vi "_PC_Pub writeListboxString.vi"(5 "Reset (F)":bool, 6 "Display Error Msg? (F)":bool, 7 "String Color":u32(colorbox), 8 "error in (no error)":errorcluster, 10 "update_Str":string, 11 "Listbox Ref Input":refnum<vi>) -> (0 "error out":errorcluster, 3 "Listbox Ref Output":refnum<vi>)   [LabVIEW 2018]
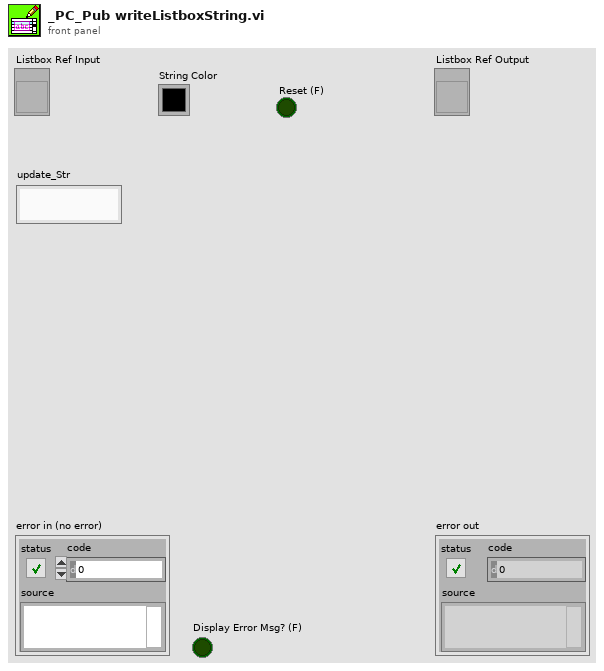
[diagram p1: front panel]
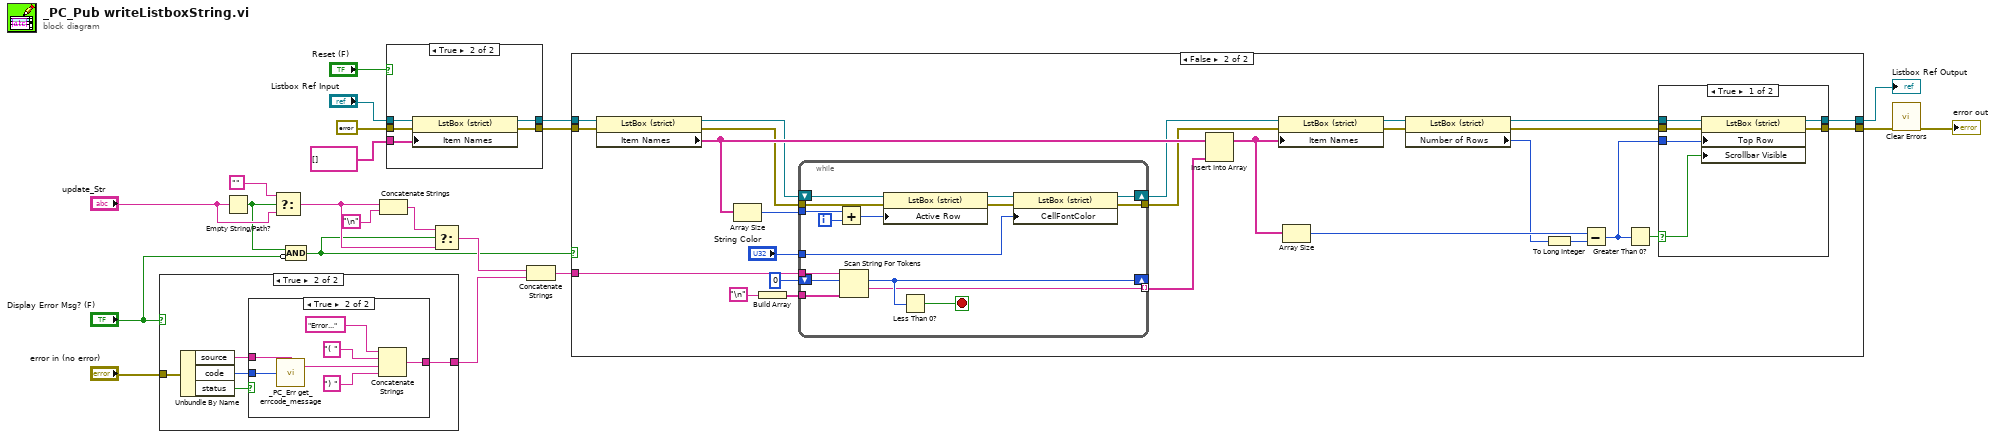
[diagram p0: block diagram]
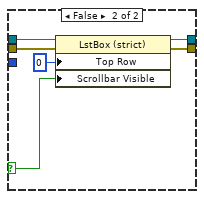
[diagram p3: hidden frame]
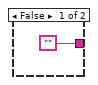
[diagram p5: hidden frame]
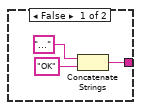
[diagram p6: hidden frame]
diagram:
  n1 = case shown="True" "Display Error Msg? (F)" {
    tunnel: "error in (no error)" -> [_ w27]
    tunnel: ["" w25] -> w21
    frame False {
    }
    frame True {
      n2 = Unbundle By Name(w27) -> ("source"=w23:string, "code"=w24:i32, "status"=w26:bool)
      n3 = case shown="True" w26 {
        tunnel: [w28 w35] -> w25
        tunnel: w24 -> [_ w33]
        tunnel: w23 -> [_ w31]
        frame False {
          n4 = Concatenate Strings("...", "OK") -> (w28:string)
        }
        frame True {
          n5 = call "_PC_Err get_errcode_message.vi"("err code"=w33, "sourceError"=w31) -> ("err msg"=w32:string)  [unwired: 1 out]
          n6 = Concatenate Strings("Error...", "( " ("string"), w32, ") " ("string")) -> (w35:string)
        }
      }
    }
  }
  n7 = Empty String/Path?(string/path="update_Str") -> (empty?=w11:bool)
  n8 = Select(t="", s=w11, f="update_Str") -> (s? t:f=w9:string)
  n9 = Compound Arithmetic op=AND(w11, invert "Display Error Msg? (F)") -> (w6:bool)
  n10 = Concatenate Strings(w9, "\n") -> (w8:string)
  n11 = case shown="True" "Reset (F)" {
    tunnel: "Listbox Ref Input" -> [w39 w44]
    tunnel: [w39 w43] -> w18
    tunnel: string[] [] ("appended array") -> [_ w42]
    tunnel: errorcluster {"status"=FALSE, "code"=0, "source"=""} ("error in (no error)") -> [w38 w41]
    tunnel: [w38 w40] -> w15
    frame False {
    }
    frame True {
      n12 = property class="LstBox (strict)"(reference=w44, error in=w41, "Item Names"=w42) -> (reference out=w43:refnum<vi>, error out=w40:errorcluster)
    }
  }
  n13 = Select(t=w8, s=w6, f=w9) -> (s? t:f=w7:string)
  n14 = Concatenate Strings(w7, w21) -> (w14:string)
  n15 = case shown="False" w6 {
    tunnel: w14 -> [_ w72]
    tunnel: w18 -> [w46 w68]
    tunnel: [w46 w60] -> w4
    tunnel: [w45 w59] -> w1
    tunnel: w15 -> [w45 w62]
    frame True {
    }
    frame False {
      n16 = property class="LstBox (strict)"(reference=w68, error in=w62) -> (reference out=w53:refnum<vi>, error out=w52:errorcluster, "Item Names"=w58:string[])
      n17 = Array Size(array=w58) -> (size(s)=w54:i32)
      n18 = Build Array("\n") -> (w71:string[])
      n19 = while {
        tunnel: w72 -> [w100]
        tunnel: w71 -> [w95]
        tunnel: [w96] -> w64 mode=indexing
        shift-right: [w99] -> _
        shift-left: 0 -> [w98]
        tunnel: w54 -> [w92]
        tunnel: w52 -> [w93]
        shift-right: [w87] -> w51
        shift-left: w53 -> [w94]
        tunnel: [w86] -> w50
        tunnel: "String Color" -> [w85]
        i -> [w91]
        stop <- w97 stop-if-true
        n20 = Add(x=w92, y=w91) -> (x+y=w90:i32)
        n21 = Scan String For Tokens(6:w95, 8:w98, 9:w100) -> (1:w96:string, 2:w99:i32)  [unwired: 3 in, 2 out]
        n22 = property class="LstBox (strict)"(reference=w94, error in=w93, "Active Row"=w90) -> (reference out=w89:refnum<vi>, error out=w88:errorcluster)
        n23 = Less Than 0?(x=w99) -> (x < 0?=w97:bool)
        n24 = property class="LstBox (strict)"(reference=w89, error in=w88, "CellFontColor"=w85) -> (reference out=w87:refnum<vi>, error out=w86:errorcluster)
      }
      n25 = Insert Into Array(array=w58, new element=w64) -> (w63:string[])  [unwired: 1 in]
      n26 = property class="LstBox (strict)"(reference=w51, error in=w50, "Item Names"=w63) -> (reference out=w48:refnum<vi>, error out=w47:errorcluster)
      n27 = Array Size(array=w63) -> (size(s)=w61:i32)
      n28 = property class="LstBox (strict)"(reference=w48, error in=w47) -> (reference out=w57:refnum<vi>, error out=w56:errorcluster, "Number of Rows"=w55:u32)
      n29 = To Long Integer(number=w55) -> (32bit integer=w67:i32)
      n30 = Subtract(x=w61, y=w67) -> (x-y=w65:i32)
      n31 = Greater Than 0?(x=w65) -> (x > 0?=w66:bool)
      n32 = case shown="True" w66 {
        selector: w66 -> [w75 w81]
        tunnel: [w77 w83] -> w60
        tunnel: w57 -> [w78 w84]
        tunnel: w65 -> [w76 _]
        tunnel: w56 -> [w73 w80]
        tunnel: [w74 w79] -> w59
        frame True {
          n33 = property class="LstBox (strict)"(reference=w78, error in=w73, "Top Row"=w76, "Scrollbar Visible"=w75) -> (reference out=w77:refnum<vi>, error out=w74:errorcluster)
        }
        frame False {
          n34 = property class="LstBox (strict)"(reference=w84, error in=w80, "Top Row"=0, "Scrollbar Visible"=w81) -> (reference out=w83:refnum<vi>, error out=w79:errorcluster)
        }
      }
    }
  }
  "Listbox Ref Output" <- w4
  n35 = call <vilib>:"Clear Errors.vi"("error in (no error)"=w1) -> ("error out"=→"error out":errorcluster)  [unwired: 5 in, 1 out]
